vi "Wizard Decision Maker.vi"(6 "Mode":enum16{"Next", "Back"}(ring), 7 "Qref out":refnum<queue>, 8 "error in":errorcluster, 9 "Tab Control":refnum<vi>, 10 "Tab Pages Ref":refnum<vi>[](array[refnum]), 11 "Tab Control":T1(ring)=enum."Page 4") -> (0 "error out":errorcluster)   [LabVIEW 2014]
doc: "<B>Copyright</B>: (c) 2015 MHWirth. All rights reserved.\n\nThis subVI is in charge of navigation between pages while Previous and Next are pressed."
uses:
  TypeDef and Controls/QWizardMessage.ctl
  Wizard Global Variable.vi
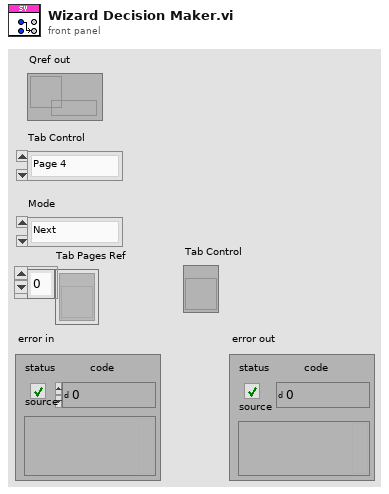
[diagram p1: front panel]
types:
  T1 = enum32{"Page 1", "Page 2", "Page 3", "Page 4", "Page 5", "Page 6", "Page 7"}
  T2 = typedef "QWizardMessage.ctl" = cluster{"State":enum16{"Initialize 0", "Initialize 1", "Initialize 2", "Initialize 3", "Initialize 4", "Back", "Next", "Check Database", "Get Lib Name", "Get Lib Folder", "Get Database", "Check Lib Availability", "Create SV Lib", "Check Binding", "Bind", "Get Processes", "Deploy", "Remove Process", "Clear Engine", "Initialize Process", "Get Process AP2", "Update Var AP2", "Import", "Redo", "Save Database", "Exit"}, "Data":variant}
  T3 = enum32{"Page 1", "Page 2", "Page 3", "Page 4", "Page 5"}
  T4 = enum32{"Page 1", "Page 2", "Page 3", "Page 4", "Page 5", "Page 6"}
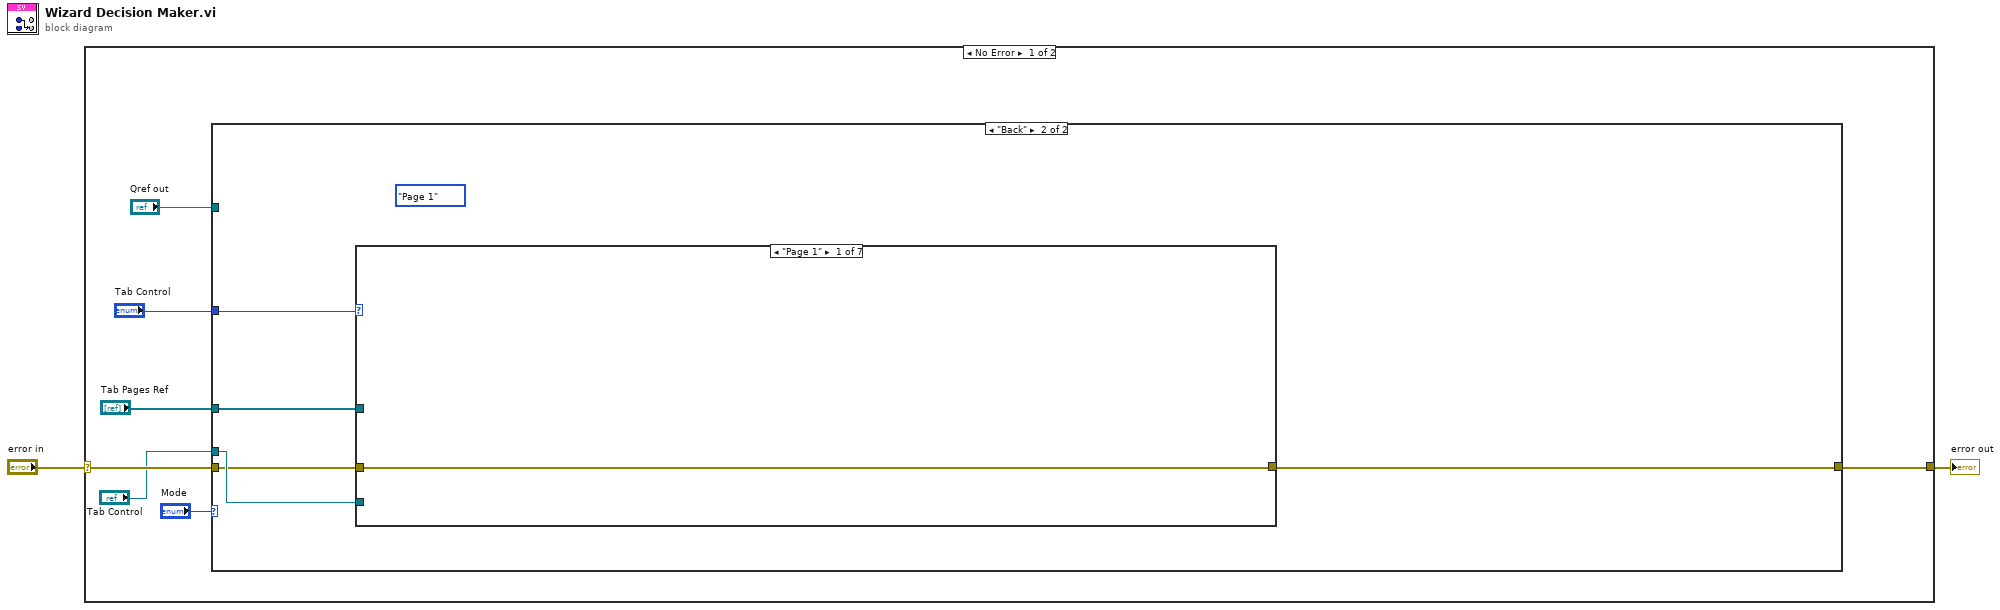
[diagram p0: block diagram]
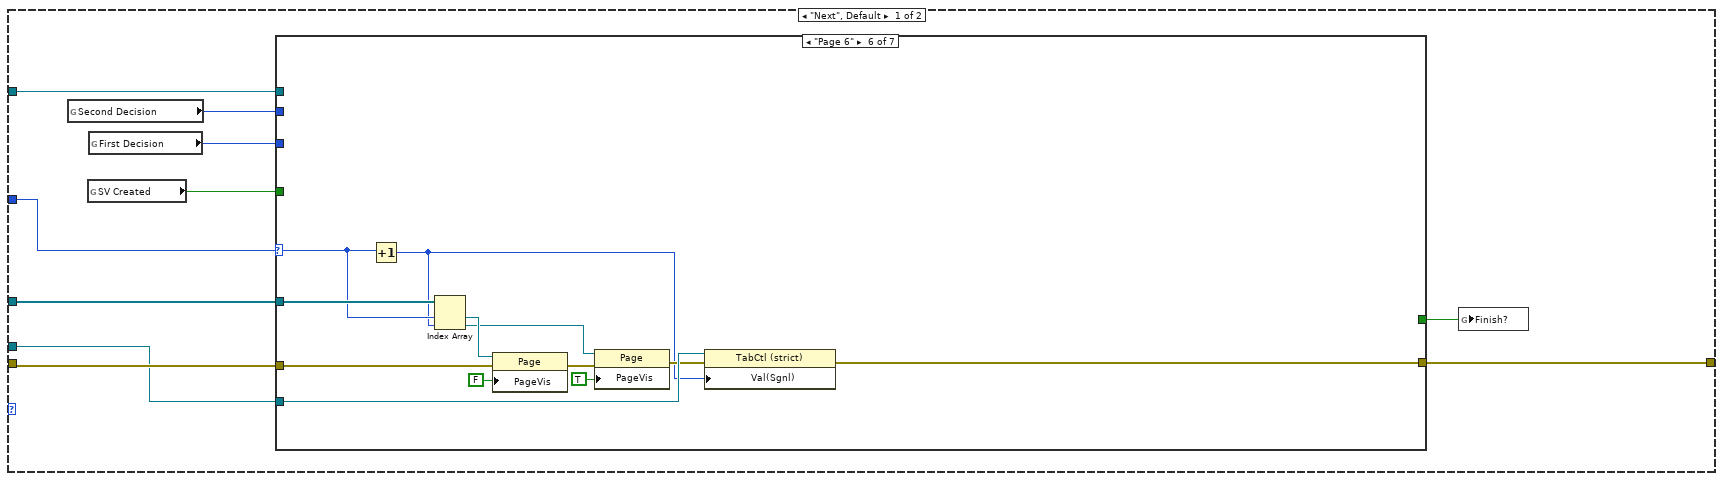
[diagram p2: hidden frame]
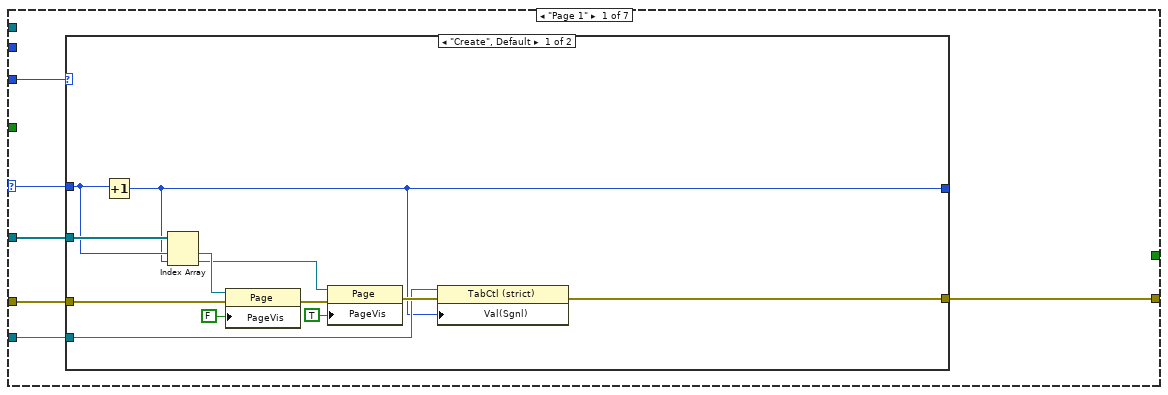
[diagram p3: hidden frame]
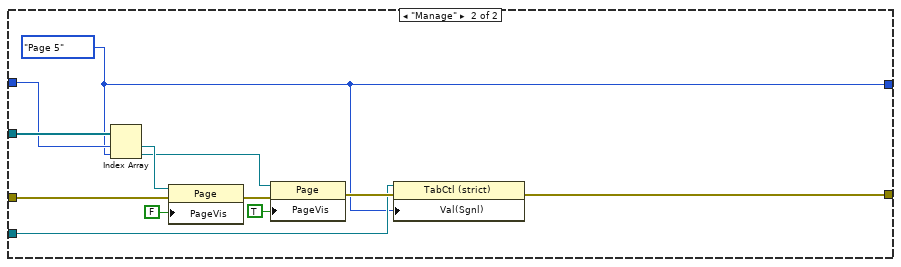
[diagram p4: hidden frame]
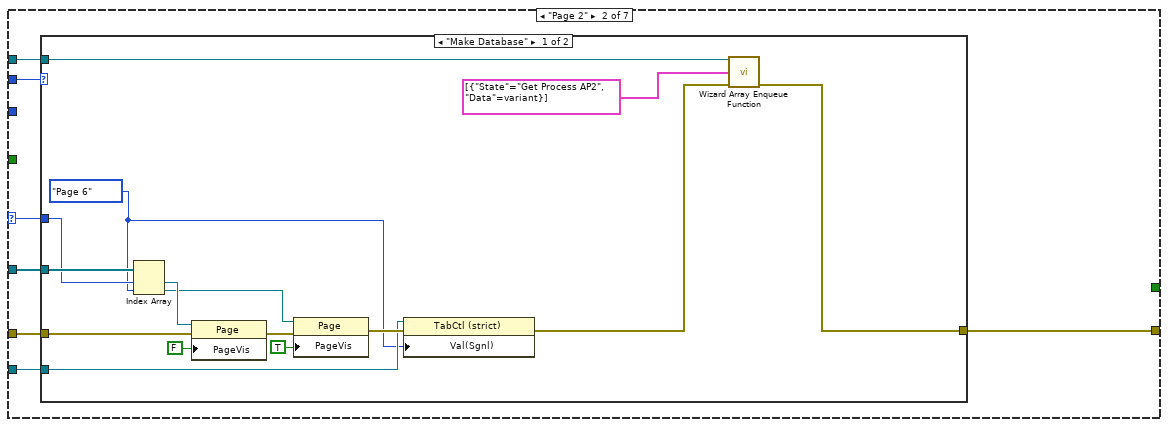
[diagram p5: hidden frame]
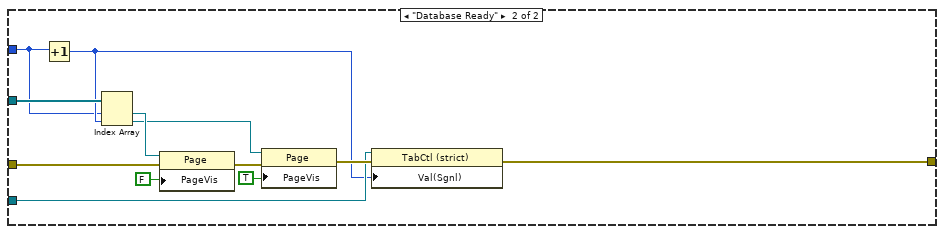
[diagram p6: hidden frame]
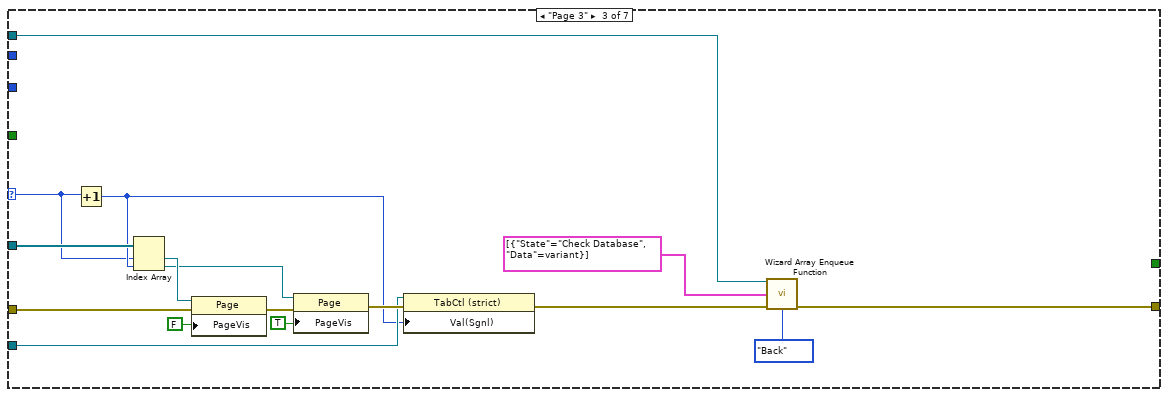
[diagram p7: hidden frame]
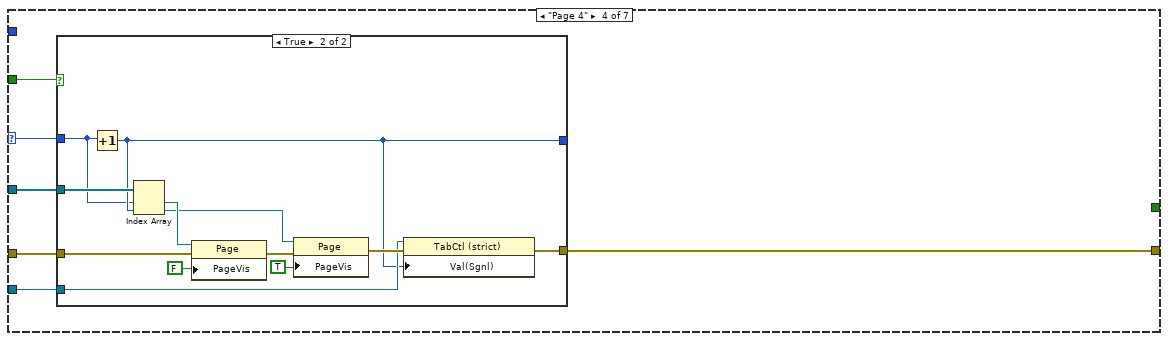
[diagram p8: hidden frame]
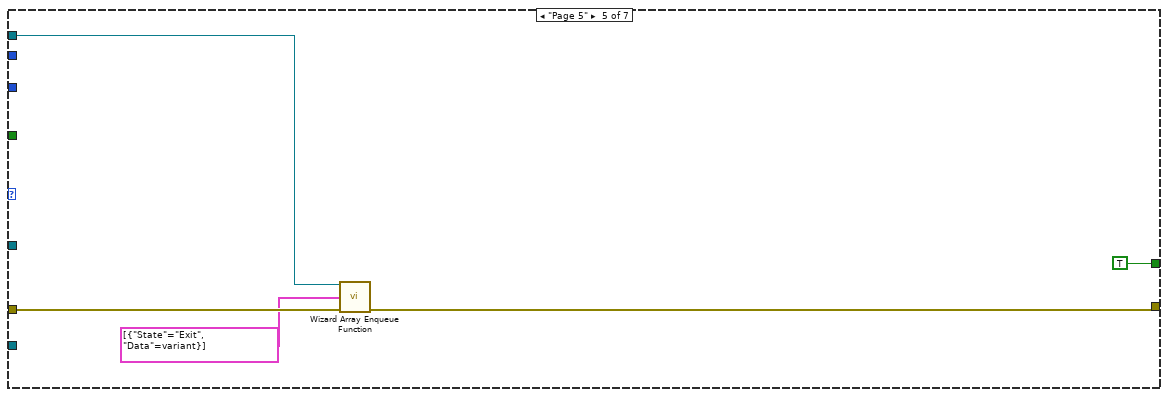
[diagram p10: hidden frame]
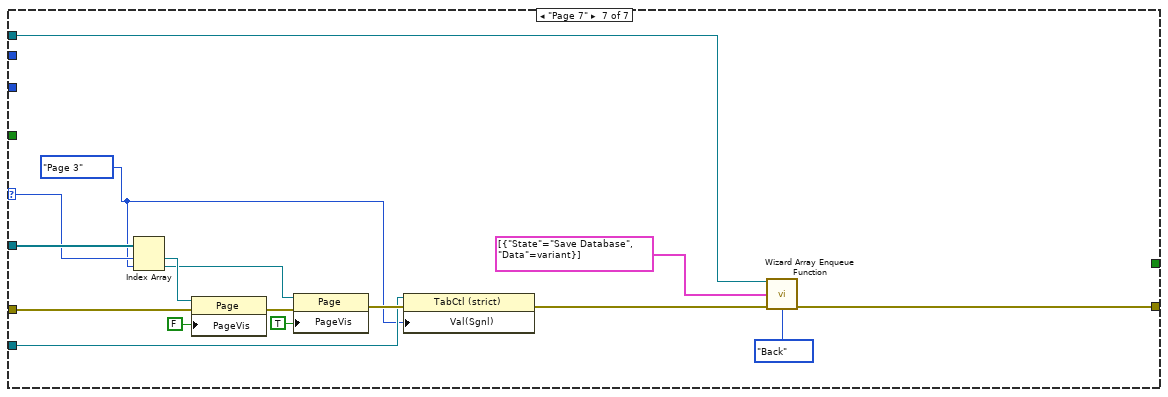
[diagram p11: hidden frame]
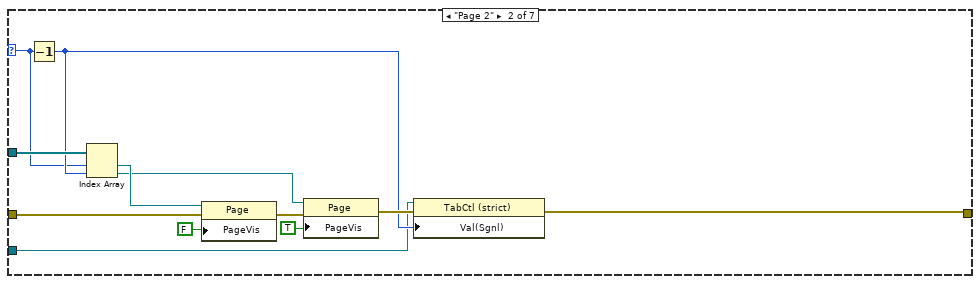
[diagram p12: hidden frame]
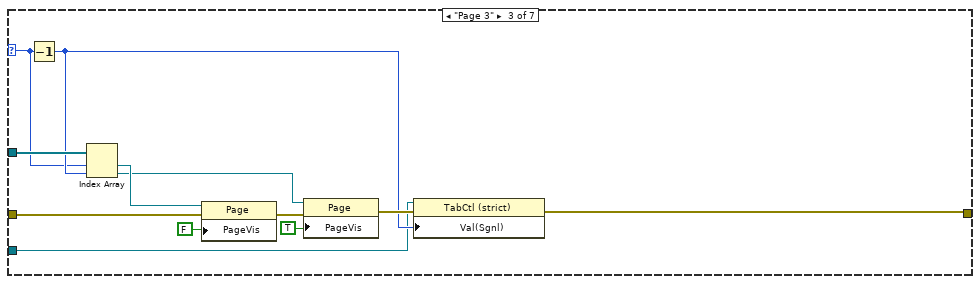
[diagram p13: hidden frame]
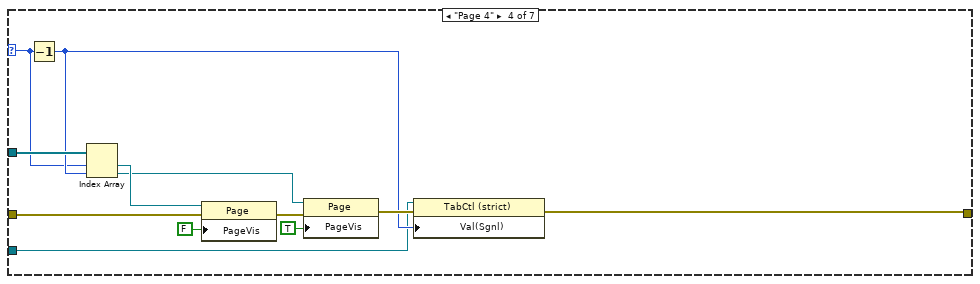
[diagram p14: hidden frame]
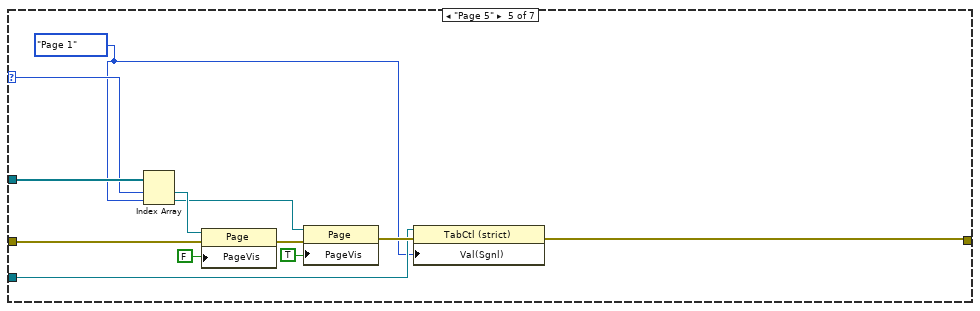
[diagram p15: hidden frame]
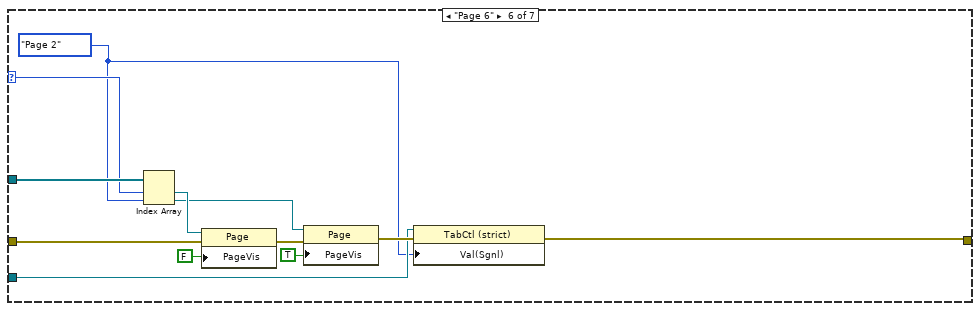
[diagram p16: hidden frame]
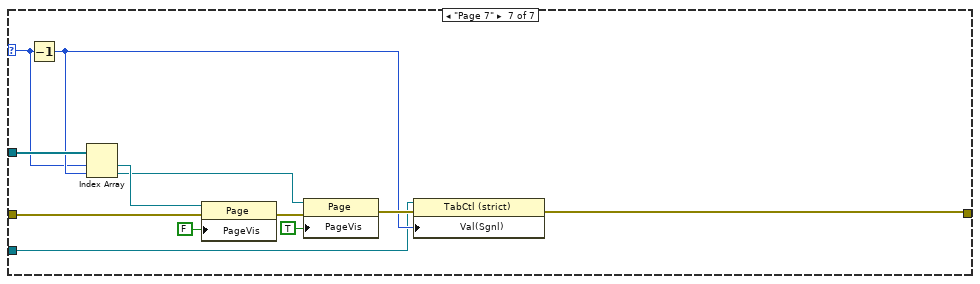
[diagram p17: hidden frame]
diagram:
  n1 = case shown="No Error" "error in" {
    selector: "error in" -> [w8 w231]
    tunnel: [w9 w231] -> w1
    frame No Error {
      n2 = case shown="\"Back\"" "Mode" {
        tunnel: "Tab Control" -> [w16 w156]
        tunnel: [w13 w153] -> w9
        tunnel: w8 -> [w18 w154]
        tunnel: "Qref out" -> [w12 _]
        tunnel: "Tab Pages Ref" -> [w19 w155]
        tunnel: "Tab Control" -> [w17 w157]
        frame "Next", Default {
          n3 = global read "Wizard Global Variable.vi" "Second Decision"() -> (w10:enum32{"Database Ready", "Make Database"})
          n4 = global read "Wizard Global Variable.vi" "SV Created"() -> (w15:bool)
          n5 = global read "Wizard Global Variable.vi" "First Decision"() -> (w14:enum32{"Create", "Manage"})
          n6 = case shown="\"Page 6\"" w16 {
            selector: w16 -> [w21 w52 w89 w101 _ w132 w143]
            tunnel: w19 -> [w25 w56 w93 w105 _ w136 w146]
            tunnel: w18 -> [w24 w55 w92 w104 w124 w135 w145]
            tunnel: w17 -> [w23 w54 w91 w103 _ w134 w144]
            tunnel: [w22 w53 w87 w102 w123 w133 w141] -> w13
            tunnel: w15 -> [_ _ _ w100 _ _ _]
            tunnel: w14 -> [w20 _ _ _ _ _ _]
            tunnel: w12 -> [_ w50 w85 _ w122 _ w139]
            tunnel: [_ _ _ _ TRUE _ _] -> w11
            tunnel: w10 -> [_ w51 _ _ _ _ _]
            frame "Page 1" {
              n7 = case shown="\"Create\", Default" w20 {
                tunnel: w25 -> [w31 w43]
                tunnel: w24 -> [w30 w42]
                tunnel: w23 -> [w29 w41]
                tunnel: [w26 w38] -> _
                tunnel: [w28 w40] -> w22
                tunnel: w21 -> [w27 w39]
                frame "Create", Default {
                  n8 = Increment(x=w27) -> (x+1=w26:T1)
                  n9 = Index Array(array=w31, index #1=w27, index #2=w26) -> (element #1=w37:refnum<vi>, element #2=w34:refnum<vi>)
                  n10 = property class="Page"(reference=w37, error in=w30, "PageVis"=FALSE ("Page Visible")) -> (error out=w35:errorcluster)  [unwired: 1 out]
                  n11 = property class="Page"(reference=w34, error in=w35, "PageVis"=TRUE ("Page Visible")) -> (error out=w32:errorcluster)  [unwired: 1 out]
                  n12 = property on="Property Node" class="TabCtl (strict)"(reference=w29, error in=w32, "Val(Sgnl)"=w26) -> (error out=w28:errorcluster)  [unwired: 1 out]
                }
                frame "Manage" {
                  w38 = T3."Page 5" ("Tab")
                  n13 = Index Array(array=w43, index #1=w39, index #2=w38) -> (element #1=w49:refnum<vi>, element #2=w46:refnum<vi>)
                  n14 = property class="Page"(reference=w49, error in=w42, "PageVis"=FALSE ("Page Visible")) -> (error out=w47:errorcluster)  [unwired: 1 out]
                  n15 = property class="Page"(reference=w46, error in=w47, "PageVis"=TRUE ("Page Visible")) -> (error out=w44:errorcluster)  [unwired: 1 out]
                  n16 = property on="Property Node" class="TabCtl (strict)"(reference=w41, error in=w44, "Val(Sgnl)"=w38) -> (error out=w40:errorcluster)  [unwired: 1 out]
                }
              }
            }
            frame "Page 2" {
              n17 = case shown="\"Make Database\"" w51 {
                tunnel: w56 -> [w65 w77]
                tunnel: w55 -> [w64 w76]
                tunnel: w54 -> [w63 w75]
                tunnel: [w58 w73] -> w53
                tunnel: w52 -> [w62 w72]
                tunnel: w50 -> [w60 _]
                frame "Make Database" {
                  w61 = T4."Page 6" ("Tab")
                  n18 = Index Array(array=w65, index #1=w62, index #2=w61) -> (element #1=w71:refnum<vi>, element #2=w68:refnum<vi>)
                  n19 = property class="Page"(reference=w71, error in=w64, "PageVis"=FALSE ("Page Visible")) -> (error out=w69:errorcluster)  [unwired: 1 out]
                  n20 = property class="Page"(reference=w68, error in=w69, "PageVis"=TRUE ("Page Visible")) -> (error out=w66:errorcluster)  [unwired: 1 out]
                  n21 = property on="Property Node" class="TabCtl (strict)"(reference=w63, error in=w66, "Val(Sgnl)"=w61) -> (error out=w59:errorcluster)  [unwired: 1 out]
                  n22 = call "Wizard Array Enqueue Function.vi"("Qref in"=w60, "Array of Messages"=T2[] [{"State"=enum."Get Process AP2", "Data"=variant}], "Error in"=w59) -> ("Error out"=w58:errorcluster)  [unwired: 11 in, 1 out]
                }
                frame "Database Ready" {
                  n23 = Increment(x=w72) -> (x+1=w74:T1)
                  n24 = Index Array(array=w77, index #1=w72, index #2=w74) -> (element #1=w83:refnum<vi>, element #2=w80:refnum<vi>)
                  n25 = property class="Page"(reference=w83, error in=w76, "PageVis"=FALSE ("Page Visible")) -> (error out=w81:errorcluster)  [unwired: 1 out]
                  n26 = property class="Page"(reference=w80, error in=w81, "PageVis"=TRUE ("Page Visible")) -> (error out=w78:errorcluster)  [unwired: 1 out]
                  n27 = property on="Property Node" class="TabCtl (strict)"(reference=w75, error in=w78, "Val(Sgnl)"=w74) -> (error out=w73:errorcluster)  [unwired: 1 out]
                }
              }
            }
            frame "Page 3" {
              n28 = Increment(x=w89) -> (x+1=w90:T1)
              n29 = Index Array(array=w93, index #1=w89, index #2=w90) -> (element #1=w99:refnum<vi>, element #2=w96:refnum<vi>)
              n30 = property class="Page"(reference=w99, error in=w92, "PageVis"=FALSE ("Page Visible")) -> (error out=w97:errorcluster)  [unwired: 1 out]
              n31 = property class="Page"(reference=w96, error in=w97, "PageVis"=TRUE ("Page Visible")) -> (error out=w94:errorcluster)  [unwired: 1 out]
              n32 = property on="Property Node" class="TabCtl (strict)"(reference=w91, error in=w94, "Val(Sgnl)"=w90) -> (error out=w88:errorcluster)  [unwired: 1 out]
              n33 = call "Wizard Array Enqueue Function.vi"("Qref in"=w85, "Array of Messages"=T2[] [{"State"=enum."Check Database", "Data"=variant}], "Error in"=w88, "Mode"=enum16{"Back", "Front", "Replace"}."Back") -> ("Error out"=w87:errorcluster)  [unwired: 10 in, 1 out]
            }
            frame "Page 4" {
              n34 = case shown="True" w100 {
                tunnel: w105 -> [_ w113]
                tunnel: w104 -> [w106 w112]
                tunnel: w103 -> [_ w111]
                tunnel: [w107 w110] -> _
                tunnel: [w106 w109] -> w102
                tunnel: w101 -> [w107 w108]
                frame False {
                }
                frame True {
                  n35 = Increment(x=w108) -> (x+1=w110:T1)
                  n36 = Index Array(array=w113, index #1=w108, index #2=w110) -> (element #1=w119:refnum<vi>, element #2=w116:refnum<vi>)
                  n37 = property class="Page"(reference=w119, error in=w112, "PageVis"=FALSE ("Page Visible")) -> (error out=w117:errorcluster)  [unwired: 1 out]
                  n38 = property class="Page"(reference=w116, error in=w117, "PageVis"=TRUE ("Page Visible")) -> (error out=w114:errorcluster)  [unwired: 1 out]
                  n39 = property on="Property Node" class="TabCtl (strict)"(reference=w111, error in=w114, "Val(Sgnl)"=w110) -> (error out=w109:errorcluster)  [unwired: 1 out]
                }
              }
            }
            frame "Page 5" {
              n40 = call "Wizard Array Enqueue Function.vi"("Qref in"=w122, "Array of Messages"=T2[] [{"State"=enum."Exit", "Data"=variant}], "Error in"=w124) -> ("Error out"=w123:errorcluster)  [unwired: 11 in, 1 out]
            }
            frame "Page 6" {
              n41 = Increment(x=w132) -> (x+1=w125:T1)
              n42 = Index Array(array=w136, index #1=w132, index #2=w125) -> (element #1=w131:refnum<vi>, element #2=w128:refnum<vi>)
              n43 = property class="Page"(reference=w131, error in=w135, "PageVis"=FALSE ("Page Visible")) -> (error out=w129:errorcluster)  [unwired: 1 out]
              n44 = property class="Page"(reference=w128, error in=w129, "PageVis"=TRUE ("Page Visible")) -> (error out=w126:errorcluster)  [unwired: 1 out]
              n45 = property on="Property Node" class="TabCtl (strict)"(reference=w134, error in=w126, "Val(Sgnl)"=w125) -> (error out=w133:errorcluster)  [unwired: 1 out]
            }
            frame "Page 7" {
              w137 = T1."Page 3" ("Tab")
              n46 = Index Array(array=w146, index #1=w143, index #2=w137) -> (element #1=w152:refnum<vi>, element #2=w149:refnum<vi>)
              n47 = property class="Page"(reference=w152, error in=w145, "PageVis"=FALSE ("Page Visible")) -> (error out=w150:errorcluster)  [unwired: 1 out]
              n48 = property class="Page"(reference=w149, error in=w150, "PageVis"=TRUE ("Page Visible")) -> (error out=w147:errorcluster)  [unwired: 1 out]
              n49 = property on="Property Node" class="TabCtl (strict)"(reference=w144, error in=w147, "Val(Sgnl)"=w137) -> (error out=w142:errorcluster)  [unwired: 1 out]
              n50 = call "Wizard Array Enqueue Function.vi"("Qref in"=w139, "Array of Messages"=T2[] [{"State"=enum."Save Database", "Data"=variant}], "Error in"=w142, "Mode"=enum16{"Back", "Front", "Replace"}."Back") -> ("Error out"=w141:errorcluster)  [unwired: 10 in, 1 out]
            }
          }
          n51 = global write "Wizard Global Variable.vi" "Finish?"(w11) -> ()
        }
        frame "Back" {
          (unwired) T1."Page 1" ("Tab Control")
          n52 = case shown="\"Page 1\"" w156 {
            selector: w156 -> [_ w160 w172 w184 w197 w209 w220]
            tunnel: w155 -> [_ w170 w182 w194 w206 w218 w230]
            tunnel: w154 -> [w158 w162 w174 w186 w199 w211 w222]
            tunnel: [w158 w161 w173 w185 w198 w210 w221] -> w153
            tunnel: w157 -> [_ w159 w171 w183 w196 w208 w219]
            frame "Page 1" {
            }
            frame "Page 2" {
              n53 = Decrement(x=w160) -> (x-1=w163:T1)
              n54 = Index Array(array=w170, index #1=w160, index #2=w163) -> (element #1=w169:refnum<vi>, element #2=w166:refnum<vi>)
              n55 = property class="Page"(reference=w169, error in=w162, "PageVis"=FALSE ("Page Visible")) -> (error out=w167:errorcluster)  [unwired: 1 out]
              n56 = property class="Page"(reference=w166, error in=w167, "PageVis"=TRUE ("Page Visible")) -> (error out=w164:errorcluster)  [unwired: 1 out]
              n57 = property on="Property Node" class="TabCtl (strict)"(reference=w159, error in=w164, "Val(Sgnl)"=w163) -> (error out=w161:errorcluster)  [unwired: 1 out]
            }
            frame "Page 3" {
              n58 = Decrement(x=w172) -> (x-1=w175:T1)
              n59 = Index Array(array=w182, index #1=w172, index #2=w175) -> (element #1=w181:refnum<vi>, element #2=w178:refnum<vi>)
              n60 = property class="Page"(reference=w181, error in=w174, "PageVis"=FALSE ("Page Visible")) -> (error out=w179:errorcluster)  [unwired: 1 out]
              n61 = property class="Page"(reference=w178, error in=w179, "PageVis"=TRUE ("Page Visible")) -> (error out=w176:errorcluster)  [unwired: 1 out]
              n62 = property on="Property Node" class="TabCtl (strict)"(reference=w171, error in=w176, "Val(Sgnl)"=w175) -> (error out=w173:errorcluster)  [unwired: 1 out]
            }
            frame "Page 4" {
              n63 = Decrement(x=w184) -> (x-1=w187:T1)
              n64 = Index Array(array=w194, index #1=w184, index #2=w187) -> (element #1=w193:refnum<vi>, element #2=w190:refnum<vi>)
              n65 = property class="Page"(reference=w193, error in=w186, "PageVis"=FALSE ("Page Visible")) -> (error out=w191:errorcluster)  [unwired: 1 out]
              n66 = property class="Page"(reference=w190, error in=w191, "PageVis"=TRUE ("Page Visible")) -> (error out=w188:errorcluster)  [unwired: 1 out]
              n67 = property on="Property Node" class="TabCtl (strict)"(reference=w183, error in=w188, "Val(Sgnl)"=w187) -> (error out=w185:errorcluster)  [unwired: 1 out]
            }
            frame "Page 5" {
              w195 = T1."Page 1" ("Tab Control")
              n68 = Index Array(array=w206, index #1=w197, index #2=w195) -> (element #1=w205:refnum<vi>, element #2=w202:refnum<vi>)
              n69 = property class="Page"(reference=w205, error in=w199, "PageVis"=FALSE ("Page Visible")) -> (error out=w203:errorcluster)  [unwired: 1 out]
              n70 = property class="Page"(reference=w202, error in=w203, "PageVis"=TRUE ("Page Visible")) -> (error out=w200:errorcluster)  [unwired: 1 out]
              n71 = property on="Property Node" class="TabCtl (strict)"(reference=w196, error in=w200, "Val(Sgnl)"=w195) -> (error out=w198:errorcluster)  [unwired: 1 out]
            }
            frame "Page 6" {
              w207 = T1."Page 2" ("Tab Control")
              n72 = Index Array(array=w218, index #1=w209, index #2=w207) -> (element #1=w217:refnum<vi>, element #2=w214:refnum<vi>)
              n73 = property class="Page"(reference=w217, error in=w211, "PageVis"=FALSE ("Page Visible")) -> (error out=w215:errorcluster)  [unwired: 1 out]
              n74 = property class="Page"(reference=w214, error in=w215, "PageVis"=TRUE ("Page Visible")) -> (error out=w212:errorcluster)  [unwired: 1 out]
              n75 = property on="Property Node" class="TabCtl (strict)"(reference=w208, error in=w212, "Val(Sgnl)"=w207) -> (error out=w210:errorcluster)  [unwired: 1 out]
            }
            frame "Page 7" {
              n76 = Decrement(x=w220) -> (x-1=w223:T1)
              n77 = Index Array(array=w230, index #1=w220, index #2=w223) -> (element #1=w229:refnum<vi>, element #2=w226:refnum<vi>)
              n78 = property class="Page"(reference=w229, error in=w222, "PageVis"=FALSE ("Page Visible")) -> (error out=w227:errorcluster)  [unwired: 1 out]
              n79 = property class="Page"(reference=w226, error in=w227, "PageVis"=TRUE ("Page Visible")) -> (error out=w224:errorcluster)  [unwired: 1 out]
              n80 = property on="Property Node" class="TabCtl (strict)"(reference=w219, error in=w224, "Val(Sgnl)"=w223) -> (error out=w221:errorcluster)  [unwired: 1 out]
            }
          }
        }
      }
    }
    frame Error {
    }
  }
  "error out" <- w1
